vi "Generate Prefixes.vi"(8 "error in (no error)":errorcluster, 10 "Groupings":T1={"Group vi.lib"=FALSE, "Group instr.lib"=FALSE, "Group user.lib"=FALSE, "Group All LabVIEW"=FALSE, "Make Custom Containers"=TRUE, "Ignore LabVIEW directory"=FALSE}, 11 "Dep Names and Paths":T2) -> (0 "error out":errorcluster, 3 "Prefixed Dep Names and Paths":T2)   [LabVIEW 2018, in "Name and Dependency Processing.lvlib"]
uses:
  Name and Dependency Processing.lvlib
  Dep Names and Paths.ctl
  Shared Dependencies/Grouping Control.ctl
  Path and string processing/Path and String Processing.lvlib
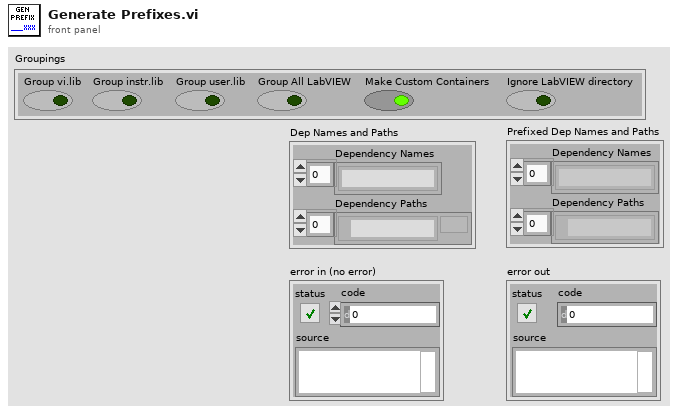
[diagram p1: front panel]
types:
  T1 = typedef "Name and Dependency Processing.lvlib/Grouping Control.ctl" = cluster{"Group vi.lib":bool, "Group instr.lib":bool, "Group user.lib":bool, "Group All LabVIEW":bool, "Make Custom Containers":bool, "Ignore LabVIEW directory":bool}
  T2 = typedef "Name and Dependency Processing.lvlib/Dep Names and Paths.ctl" = cluster{"Dependency Names":string[], "Dependency Paths":path[]}
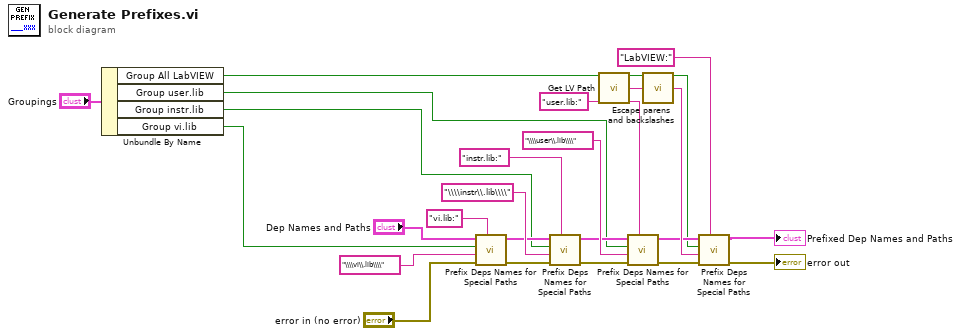
[diagram p0: block diagram]
diagram:
  n1 = Unbundle By Name("Groupings") -> ("Group All LabVIEW"=w6:bool, "Group user.lib"=w3:bool, "Group instr.lib"=w5:bool, "Group vi.lib"=w4:bool)
  n2 = call "Prefix Deps Names for Special Paths.vi"("Prefix to add"="vi.lib:" ("string"), "error in"="error in (no error)", "Regex to identify need for prefix"="\\\\vi\\.lib\\\\" ("regular expression"), "Add Prefix?"=w4, "Dep Names and Paths"="Dep Names and Paths") -> ("error out"=w20:errorcluster, "Prefixed Dep Names and Paths"=w14:T2)  [unwired: 5 in]
  n3 = call "Prefix Deps Names for Special Paths.vi"("Prefix to add"="instr.lib:" ("string"), "error in"=w20, "Regex to identify need for prefix"="\\\\instr\\.lib\\\\" ("regular expression"), "Add Prefix?"=w5, "Dep Names and Paths"=w14) -> ("error out"=w21:errorcluster, "Prefixed Dep Names and Paths"=w12:T2)  [unwired: 5 in]
  n4 = call "Get LV Path.vi"() -> ("String"=w15:string)
  n5 = call "Prefix Deps Names for Special Paths.vi"("Prefix to add"="user.lib:" ("string"), "error in"=w21, "Regex to identify need for prefix"="\\\\user\\.lib\\\\" ("regular expression"), "Add Prefix?"=w3, "Dep Names and Paths"=w12) -> ("error out"=w24:errorcluster, "Prefixed Dep Names and Paths"=w13:T2)  [unwired: 5 in]
  n6 = call "Escape parens and backslashes.vi"("Input String"=w15) -> ("Escaped String"=w23:string)  [unwired: 14 in]
  n7 = call "Prefix Deps Names for Special Paths.vi"("Prefix to add"="LabVIEW:" ("Replacement String"), "error in"=w24, "Regex to identify need for prefix"=w23, "Add Prefix?"=w6, "Dep Names and Paths"=w13) -> ("error out"=→"error out":errorcluster, "Prefixed Dep Names and Paths"=→"Prefixed Dep Names and Paths":T2)  [unwired: 5 in]
